vi "Configure Math Expression.vi"(5 "Math Expression Unit (W)":string="W", 6 "Expression Definition ((VOLT*CURR))":string="(VOLT*CURR)", 7 "Enable Math Expression (F: Disable)":bool, 8 "error in (no error)":errorcluster, 9 "Expression Name (MyMath1)":string="MyMath1", 10 "Channel (1: Channel 1)":i32(ring)=1 items=["Channel 1"=1, "Channel 2"=2], 11 "VISA resource name":refnum<visa-resource-name>) -> (0 "error out":errorcluster, 3 "VISA resource name out":refnum<visa-resource-name>)   [LabVIEW 2012, in "Keysight B2980 Series.lvlib"]
doc: "Defines a math expression to perform the Limit Test Calculation."
uses:
  Keysight B2980 Series.lvlib
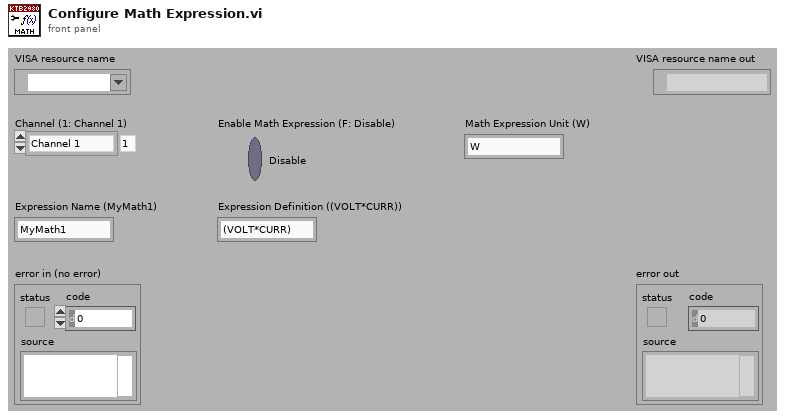
[diagram p1: front panel]
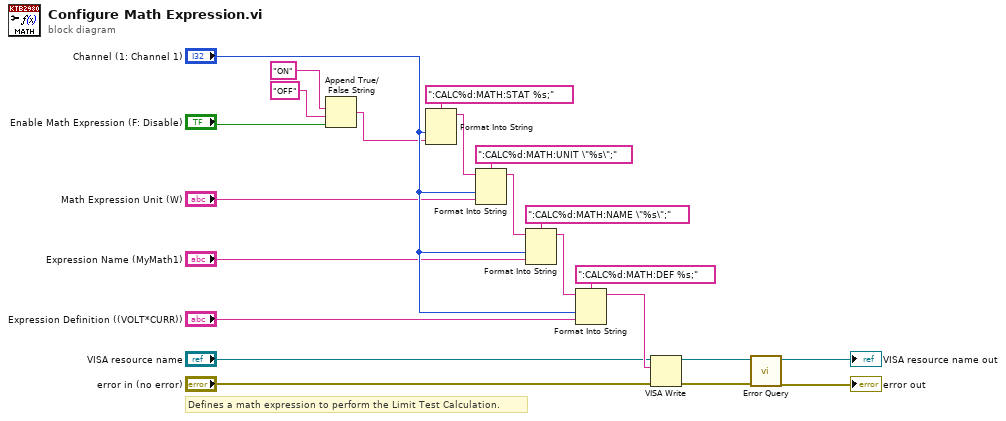
[diagram p0: block diagram]
diagram:
  # "Defines a math expression to perform the Limit Test Calculation."
  n1 = Append True/False String(1:"Enable Math Expression (F: Disable)", 2:"OFF", 3:"ON") -> (0:w17:string)  [unwired: 1 out]
  n2 = Format Into String(format string=":CALC%d:MATH:STAT %s;", "Channel (1: Channel 1)", w17) -> (resulting string=w16:string)  [unwired: 2 in, 1 out]
  n3 = Format Into String(format string=":CALC%d:MATH:UNIT \"%s\";", initial string=w16, "Channel (1: Channel 1)", "Math Expression Unit (W)") -> (resulting string=w13:string)  [unwired: 1 in, 1 out]
  n4 = Format Into String(format string=":CALC%d:MATH:NAME \"%s\";", initial string=w13, "Channel (1: Channel 1)", "Expression Name (MyMath1)") -> (resulting string=w10:string)  [unwired: 1 in, 1 out]
  n5 = Format Into String(format string=":CALC%d:MATH:DEF %s;", initial string=w10, "Channel (1: Channel 1)", "Expression Definition ((VOLT*CURR))") -> (resulting string=w7:string)  [unwired: 1 in, 1 out]
  n6 = VISA Write(VISA resource name="VISA resource name", write buffer=w7, error in (no error)="error in (no error)") -> (VISA resource name out=w4:refnum<visa-resource-name>, error out=w3:errorcluster)  [unwired: 1 out]
  n7 = call "Error Query.vi"("error in (no error)"=w3, "VISA resource name"=w4) -> ("error out"=→"error out":errorcluster, "VISA resource name out"=→"VISA resource name out":refnum<visa-resource-name>)  [unwired: 8 out]
